vi "Reset stop loops flag.vi"(8 "error in (no error)":errorcluster) -> (0 "error out":errorcluster)   [LabVIEW 2020, in "global_stop_flag.lvlib"]
uses:
  global_stop_flag.lvlib
panel:
  # "Development\ncontrols/indicators useful for development and testing, but which are not outputs of the VI"
  # "Input\nInputs to the VI"
  # "Output\nOutputs of the VI"
  # "Description\n\nBlank VI with error handling case. \n\nSummarize the use of this VI in this space."
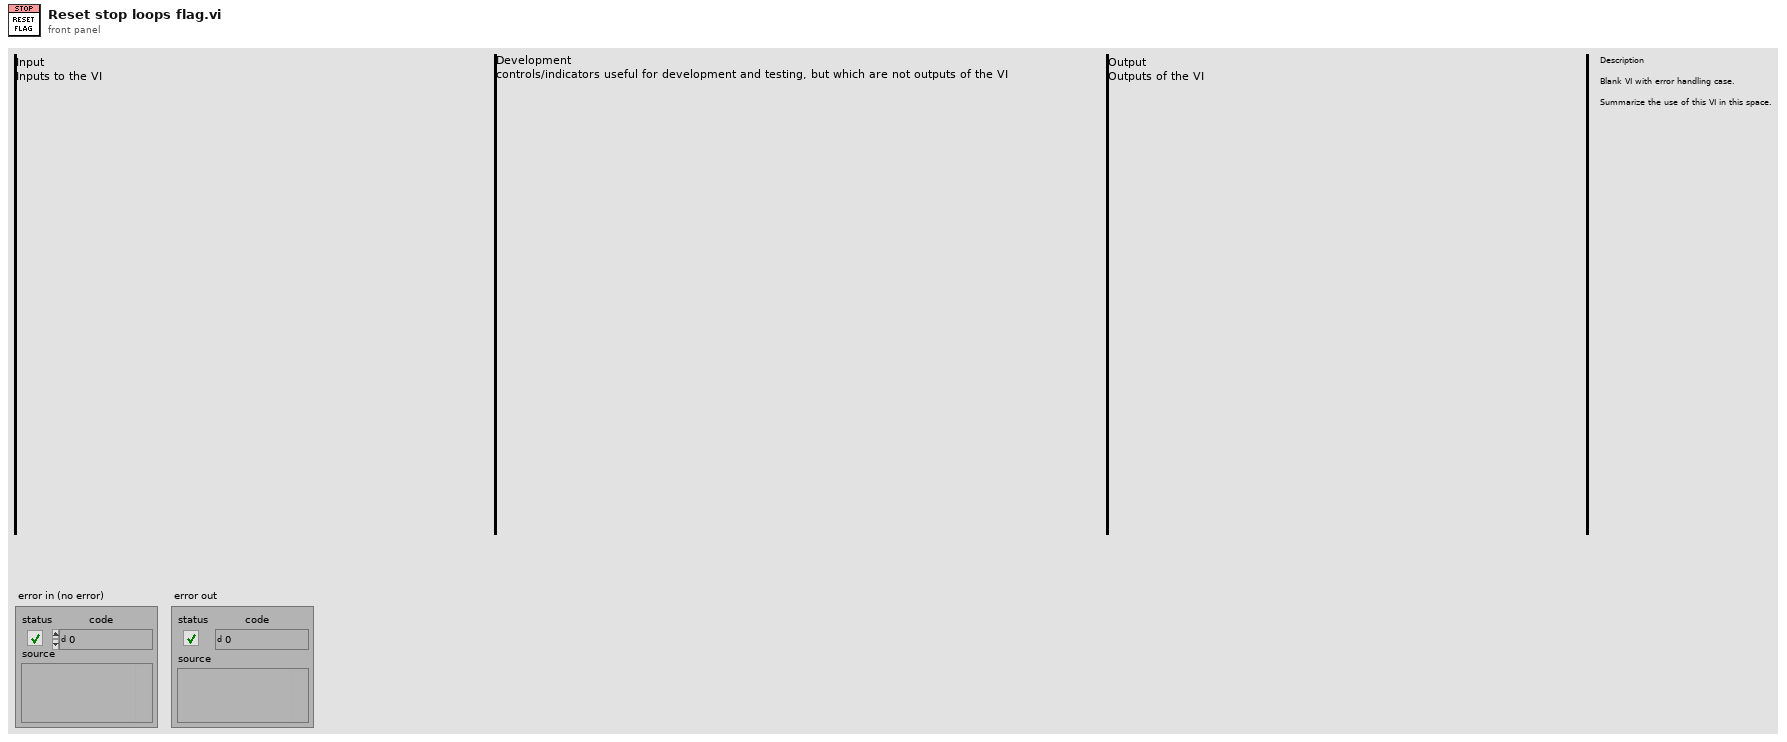
[diagram p1: front panel]
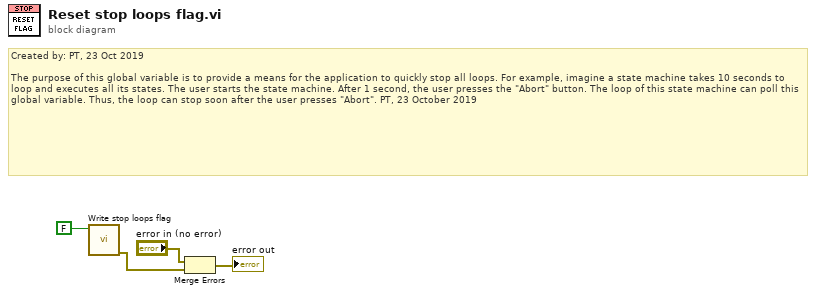
[diagram p0: block diagram]
diagram:
  # "Created by: PT, 23 Oct 2019\n\nThe purpose of this global variable is to provide a means for the application to quickly stop all loops. For example, imagine a state machine takes 10 seconds to loop and executes all its states. The user starts the state machine. After 1 second, the user presses the \"Abort\" button. The loop of this state machine can poll this global variable. Thus, the loop can stop soon after the user presses \"Abort\". PT, 23 October 2019"
  n1 = call "Write stop loops flag.vi"("Stop all loops?"=FALSE) -> ("error out"=w1:errorcluster)  [unwired: 10 in]
  n2 = Merge Errors("error in (no error)", w1) -> (→"error out":errorcluster)
